vi "move_crystal.vi"(8 "error in":errorcluster, 9 "Direction":enum16{"Reverse", "Forward"}(ring), 10 "Crystal Number":u16(ring) items=["Crystal 1", "Crystal 2", "Crystal 3", "Crystal 4", "Crystal 5", "Crystal 6", "Crystal 7", ""], 11 "address":string) -> (0 "error out":errorcluster, 2 "Crystal Number Out":u16(ring) items=["Crystal 1", "Crystal 2", "Crystal 3", "Crystal 4", "Crystal 5", "Crystal 6", "Crystal 7", ""])   [LabVIEW 2020]
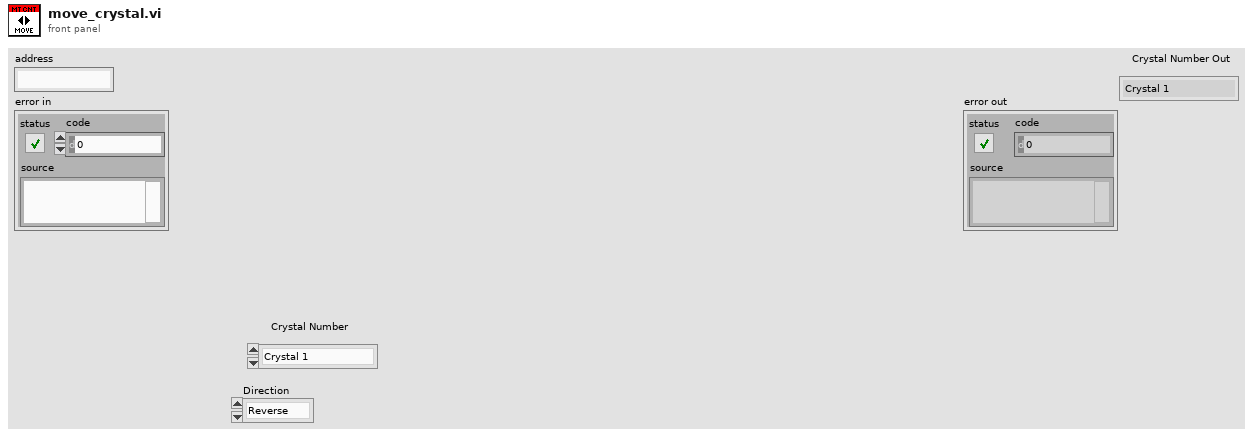
[diagram p1: front panel]
types:
  T1 = enum16{"Standard", "Buffered", "CRLF", "Immediate"}
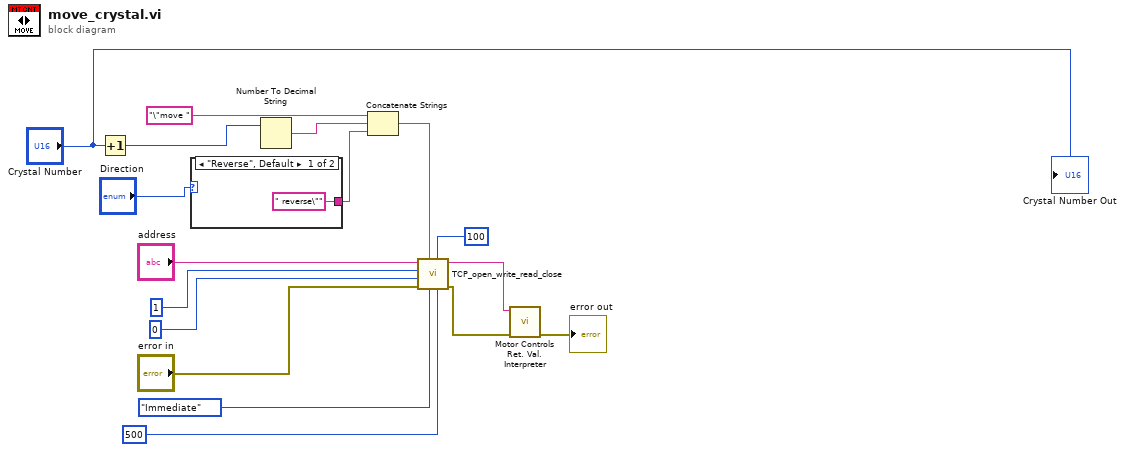
[diagram p0: block diagram]
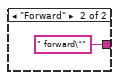
[diagram p2: hidden frame]
diagram:
  n1 = Increment(x="Crystal Number") -> (x+1=w2:u16)
  n2 = case shown="\"Reverse\", Default" "Direction" {
    tunnel: [" reverse\"" " forward\""] -> w1
    frame "Reverse", Default {
    }
    frame "Forward" {
    }
  }
  n3 = Number To Decimal String(number=w2) -> (decimal integer string=w5:string)  [unwired: 1 in]
  n4 = Concatenate Strings("\"move " ("write string"), w5, w1) -> (w11:string)
  n5 = call "TCP_open_write_read_close.vi"("timeout ms (25000)"=500, "bytes to read"=100, "mode (standard)"=T1."Immediate", "write string"=w11, "error in"="error in", "local port (0)"=u16 0, "remote port or service name"=u16 1, "address"="address") -> ("error out"=w9:errorcluster, "read string"=w7:string)  [unwired: 2 in]
  n6 = call "Motor Controls Ret. Val. Interpreter.vi"("error in"=w9, "Command Return"=w7) -> ("error out"=→"error out":errorcluster)  [unwired: 8 in, 1 out]
  "Crystal Number Out" <- "Crystal Number"
